vi "Get Optimiser Cell.vi"(8 "error in (no error)":errorcluster, 11 "Run Block in":refnum<class "Run Block.lvclass">) -> (0 "error out":errorcluster, 2 "Optimiser Cell":refnum<class "Optimiser Cell.lvclass">, 3 "Run Block out":refnum<class "Run Block.lvclass">)   [LabVIEW 2020, in "Run Utilities.lvlib" / "Run Block.lvclass"]
doc: "VI for obtaining the first cell in the schedule and casting it into optimiser cell. If the cell is not an optimser cell, this VI will throw errors"
uses:
  Run Block.lvclass
  Optimiser Cell/Optimiser Cell.lvclass
  Schedule/Schedule.lvclass
  Run Block.lvclass/Run Block.ctl
  TALOS/TALOS_PPL.lvlibp
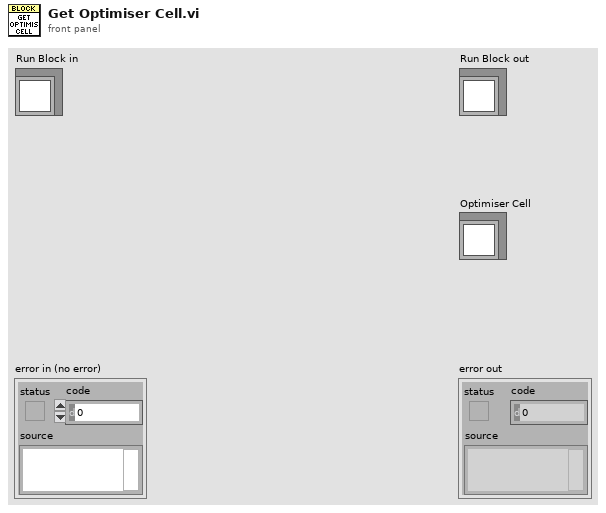
[diagram p1: front panel]
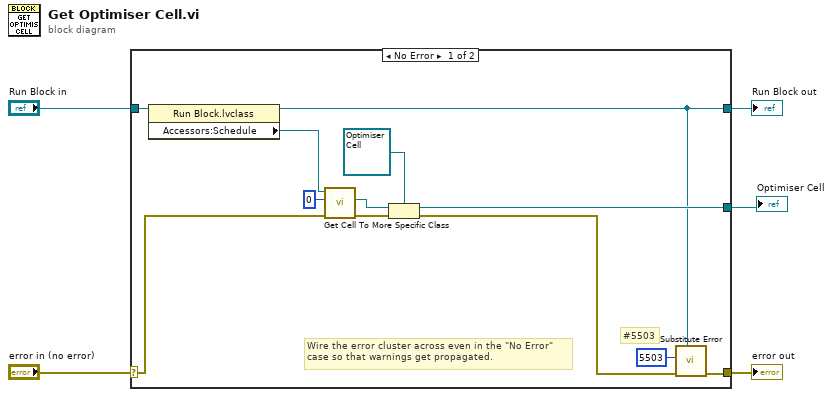
[diagram p0: block diagram]
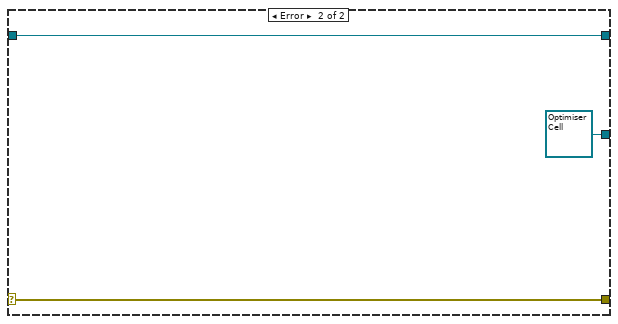
[diagram p2: hidden frame]
diagram:
  n1 = case shown="No Error" "error in (no error)" {
    selector: "error in (no error)" -> [w14 w20]
    tunnel: [w8 w20] -> w4
    tunnel: [w7 w19] -> w2
    tunnel: "Run Block in" -> [w17 w19]
    tunnel: [w10 refnum<class "Optimiser Cell.lvclass"> refnum ("Scheduling.lvlib:Optimiser Cell.lvclass")] -> w1
    frame No Error {
      # "#5503"
      # "Wire the error cluster across even in the \"No Error\"\ncase so that warnings get propagated."
      n2 = property class="Run Block.lvclass"(reference=w17) -> (reference out=w7:refnum<class "Run Block.lvclass">, "Accessors:Schedule"=w16:refnum<class "Schedule.lvclass">)  [unwired: 1 in, 1 out]
      n3 = call-dynamic "Get Cell.vi"("error in (no error)"=w14, "index"=0, "Schedule in"=w16) -> ("error out"=w12:errorcluster, "Schedule Cell"=w13:refnum<class "Schedule Cell.lvclass">)  [unwired: 6 in, 1 out]
      n4 = To More Specific Class(target class=refnum<class "Optimiser Cell.lvclass"> refnum ("Scheduling.lvlib:Optimiser Cell.lvclass"), reference=w13, error in=w12) -> (specific class reference=w10:refnum<class "Optimiser Cell.lvclass">, error out=w9:errorcluster)
      n5 = call "Substitute Error.vi"("LabVIEW Object"=w7, "error in (no error)"=w9, "Error Code"=5503) -> ("error out"=w8:errorcluster)  [unwired: 8 in]
    }
    frame Error {
    }
  }
  "error out" <- w4
  "Run Block out" <- w2
  "Optimiser Cell" <- w1
